vi "Frame.Settings.vi"(6 "Action":enum8{"Get", "Set"}(ring), 8 "error in (no error)":errorcluster, 10 "Frame.Settings":T1, 11 "Item Ref in":T2 format="%.0x") -> (0 "error out":errorcluster, 2 "Frame.Settings":T1, 3 "Item Ref out":T2 format="%.0x")   [LabVIEW 2019, in "Ghost Bus Addon System Explorer.lvlib"]
uses:
  Ghost Bus Addon System Explorer.lvlib
  <vilib>/NI VeriStand/Custom Device API/Custom Device API.lvlib
  <vilib>/NI VeriStand/Custom Device API/Get Item Property (U32).vi
  <vilib>/NI VeriStand/Custom Device API/Set Item Property (U32).vi
  Addon Shared/SubVIs/GUID Lookup.vi
  Addon Shared/Ghost Bus Addon Shared.lvlib
  <vilib>/NI VeriStand/Custom Device API/Custom Device Item Ref.ctl
  Addon Shared/Types/Frame Settings.ctl
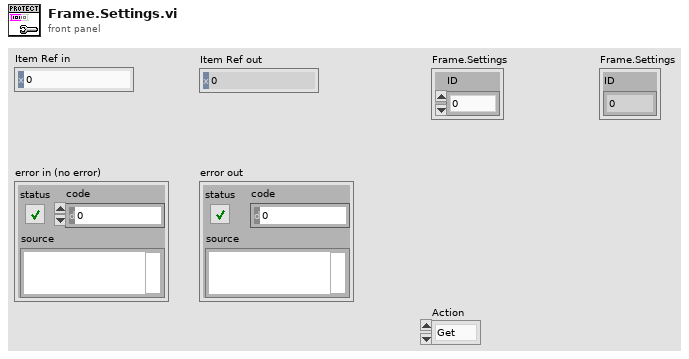
[diagram p1: front panel]
types:
  T1 = typedef "Frame Settings.ctl" = cluster{"ID":u32}
  T2 = typedef "Custom Device API.lvlib/Custom Device Item Ref.ctl" = u64
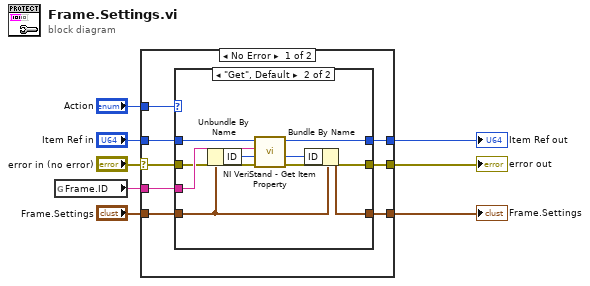
[diagram p0: block diagram]
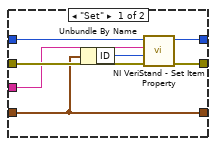
[diagram p2: hidden frame]
diagram:
  n1 = global read "GUID Lookup.vi" "Frame.ID"() -> (w1:string)
  n2 = case shown="No Error" "error in (no error)" {
    selector: "error in (no error)" -> [w11 w34]
    tunnel: "Item Ref in" -> [w16 w33]
    tunnel: w1 -> [w15 _]
    tunnel: [w14 w34] -> w7
    tunnel: [w13 w33] -> w6
    tunnel: [w12 _] -> w5
    tunnel: "Frame.Settings" -> [w10 _]
    tunnel: "Action" -> [w9 _]
    frame No Error {
      n3 = case shown="\"Get\", Default" w9 {
        tunnel: w16 -> [w23 w28]
        tunnel: w15 -> [w19 w32]
        tunnel: [w22 w27] -> w14
        tunnel: [w21 w26] -> w13
        tunnel: [w18 w30] -> w12
        tunnel: w11 -> [w20 w29]
        tunnel: w10 -> [w18 w25]
        frame "Set" {
          n4 = Unbundle By Name(w18) -> ("ID"=w17:u32)
          n5 = call-poly <vilib>:"NI VeriStand - Set Item Property.vi"("error in (no error)"=w20, "Value"=w17, "Property Name"=w19, "Item Ref in"=w23) -> ("error out"=w22:errorcluster, "Item Ref out"=w21:T2)  [unwired: 5 in, 1 out]
        }
        frame "Get", Default {
          n6 = Unbundle By Name(w25) -> ("ID"=w24:u32)
          n7 = call-poly <vilib>:"NI VeriStand - Get Item Property.vi"("error in (no error)"=w29, "Default Value"=w24, "Property Name"=w32, "Item Ref in"=w28) -> ("error out"=w27:errorcluster, "Value"=w31:u32, "Item Ref out"=w26:T2)  [unwired: 4 in, 1 out]
          n8 = Bundle By Name(cluster=w25, "ID"=w31) -> (w30:T1)
        }
      }
    }
    frame Error {
    }
  }
  "Item Ref out" <- w6
  "error out" <- w7
  "Frame.Settings" <- w5
